vi "Counter_Output.vi"(8 "error in":errorcluster caption="entrée d'erreur") -> (0 "error out":errorcluster caption="sortie d'erreur")   [LabVIEW 2026]
panel:
  in  "stop":bool
  in  "Duty Cycle":dbl(slide)=50.0 scale=0.0..100.0
  in  "F (Hz)":dbl=1000.0
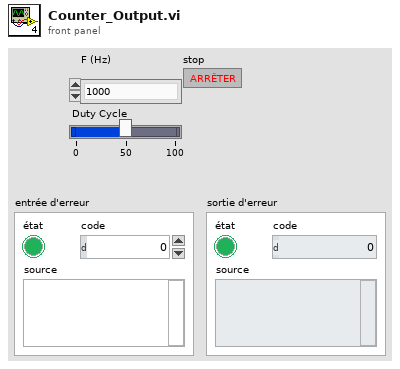
[diagram p1: front panel]
types:
  T1 = enum32{"Finite", "Continuous", "Resend One Buffer"}
  T2 = enum32{"Internal Clock", "External Clock", "No Timing"}
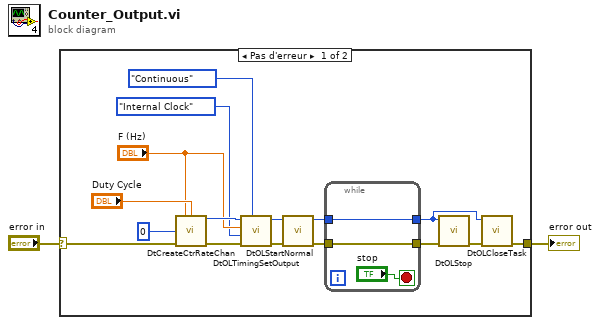
[diagram p0: block diagram]
diagram:
  n1 = case shown="Pas d'erreur" "error in" {
    selector: "error in" -> [w4 w22]
    tunnel: [w3 w22] -> w2
    frame No Error {
      n2 = call <userlib>:"DtCreateCtrRateChan.vi"("Requested\nFrequency (Hz)"="F (Hz)", "Duty Cycle"="Duty Cycle", "Counter Num"=u32 0, "error in (no error)"=w4) -> ("Task out"=w16:i32, "error out"=w15:errorcluster)  [unwired: 9 in, 1 out]
      n3 = call <userlib>:"DtOLTimingSetOutput.vi"("Sample Mode"=T1."Continuous", "error in (no error)"=w15, "Timing"=T2."Internal Clock", "Sample Freq (Hz)"="F (Hz)", "Task in"=w16) -> ("error out"=w10:errorcluster, "Task out"=w11:i32)  [unwired: 4 in, 1 out]
      n4 = call <userlib>:"DtOLStartNormal.vi"("error in (no error)"=w10, "Task in"=w11) -> ("error out"=w9:errorcluster, "Task out"=w8:i32)  [unwired: 8 in]
      n5 = while {
        tunnel: w9 -> [w20]
        tunnel: w8 -> [w19]
        tunnel: [w20] -> w5
        tunnel: [w19] -> w7
        stop <- "stop" stop-if-true
      }
      n6 = call <userlib>:"DtOLStop.vi"("error in (no error)"=w5, "Task in"=w7) -> ("error out"=w6:errorcluster)  [unwired: 8 in, 1 out]
      n7 = call <userlib>:"DtOLCloseTask.vi"("Error in"=w6, "Task in"=w7) -> ("Error Out"=w3:errorcluster)  [unwired: 9 in]
    }
    frame Error {
    }
  }
  "error out" <- w2
